vi "Single Channel FPGA C reset.vi"(5 "Reset":bool, 7 "Period (Ticks)":u32=2000, 8 "INHB":bool, 9 "DIR":bool, 10 "Duty":fxp<+,32,0>, 11 "IO Channels":T1={"PWM In"="Connector1/DIO20", "Direction"="Connector1/DIO20", "Inhibit"="Connector1/DIO20", "Encoder C"="Connector1/DIO20", "Encoder B"="Connector1/DIO20", "Encoder A"="Connector1/DIO20", "Fault"="Connector1/DIO20"}) -> (0 "FAULT":bool, 2 "JumpBy2Error":i16, 3 "Position":i32)   [LabVIEW 2016, in "jmslib.lvlib"]
uses:
  jmslib.lvlib
  <vilib>/rvi/eio/common/nirviEmuTemplateMethod_errors.vi
  <vilib>/eio/EIONode/EIONode.xnode
  KevinLibraryAll/labview2010/kevLib2010.lvlib
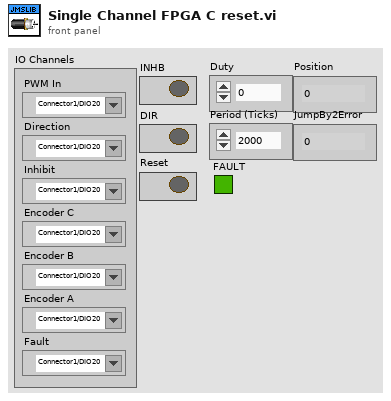
[diagram p1: front panel]
types:
  T1 = cluster{"PWM In":refnum<k21>, "Direction":refnum<k21>, "Inhibit":refnum<k21>, "Encoder C":refnum<k21>, "Encoder B":refnum<k21>, "Encoder A":refnum<k21>, "Fault":refnum<k21>}
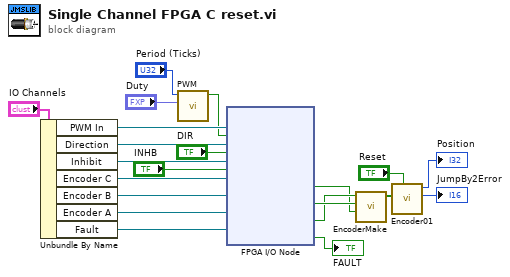
[diagram p0: block diagram]
diagram:
  n1 = Unbundle By Name("IO Channels") -> ("PWM In"=w10:refnum<k21>, "Direction"=w9:refnum<k21>, "Inhibit"=w8:refnum<k21>, "Encoder C"=w6:refnum<k21>, "Encoder B"=w5:refnum<k21>, "Encoder A"=w4:refnum<k21>, "Fault"=w3:refnum<k21>)
  n2 = call "PWM.vi"("Duty Cycle"="Duty", "Period (Ticks)"="Period (Ticks)") -> ("PWM Out"=w7:bool)  [unwired: 8 in, 1 out]
  n3 = xnode "FPGA I/O Node"("I/O Item"=w7, "FPGA I/O In"=w10, "I/O Item"="DIR", "FPGA I/O In"=w9, "I/O Item"="INHB", "FPGA I/O In"=w8, "FPGA I/O In"=w6, "FPGA I/O In"=w5, "FPGA I/O In"=w4, "FPGA I/O In"=w3) -> ("I/O Item"=w1:bool, "I/O Item"=w17:bool, "I/O Item"=w16:bool, "I/O Item"=→"FAULT":bool)  [unwired: 7 out]
  n4 = call "EncoderMake.vi"("C"=w1, "B"=w17, "A"=w16) -> ("Encoder Array"=w15:bool[])  [unwired: 8 in]
  n5 = call "Encoder01.vi"("ForceReset"="Reset", "Encoder Array"=w15) -> ("JumpBy2Error"=→"JumpBy2Error":i16, "Position"=→"Position":i32)  [unwired: 6 in, 2 out]
